vi "PV General operating info.vi"(8 "error in (no error)":errorcluster, 9 "Parameter":u16(ring) items=["nominal speed [Hz] (default) (315)", "intermediate circut current [A] (310)", "motor voltage [V] (313)", "actual power [W] (316)", "operating hours pump [h] (311)", "operating hours drive [h] (314)", "pump cycles (read only) (319)", "status oil sensor (read only) (301)", "speed switchpoint attained (read only) (302)", "overtemperature drive (read only) (304)", "overtemperature pump (read only) (305)", "target speed attained (read only) (306)", "pump accelerates (read only) (307) ", "controlled by remote (300)", "motor phase current [A] (317)", "acceleration / deceleration [rm/s] (336)", "hardware version controller (354)", "target speed (397)", "acutal speed (398)", "nominal speed (399)", "software version control unit (read only) (352)"], 10 "Adress of unit":u16=1 min=1 max=999 step=1, 11 "VISA session":refnum<visa-resource-name>) -> (0 "error out":errorcluster, 2 "response (data)":string, 3 "dup VISA session":refnum<visa-resource-name>)   [LabVIEW 2018, in "Pfeiffer Vacuum.lvlib"]
doc: "There are 21 parameters available, only one of which can be enabled at a time. \n\nnominal speed [Hz] (default) (315)\nintermediate circut current [A] (310)\nmotor voltage [V] (313)\nactual power [W] (316)\noperating hours pump [h] (311)\noperating hours drive [h] (314)\npump cycles (read only) (319)\nstatus oil sensor (read only) (301)\nspeed switchpoint attained (read only) (302)\novertemperature drive (read only) (304)\novertemperature pump (read only) (305)\ntarget speed attained (read only) (306)\npump accelerates (read only) (307)\ncontrolled by remote (300)\nmotor phase current [A] (317)\nacceleration / deceleration [rm/s] (336)\nhardware version controller (354)\ntarget speed (397)\nacutal speed (398)\nnominal speed (399)\nsoftware version control unit (read only) (352)\n\nNote: read only VI´s"
uses:
  Pfeiffer Vacuum.lvlib
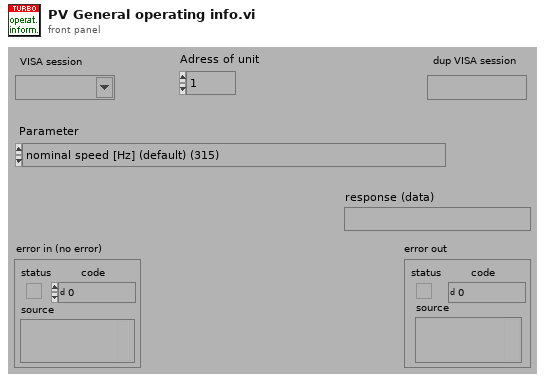
[diagram p1: front panel]
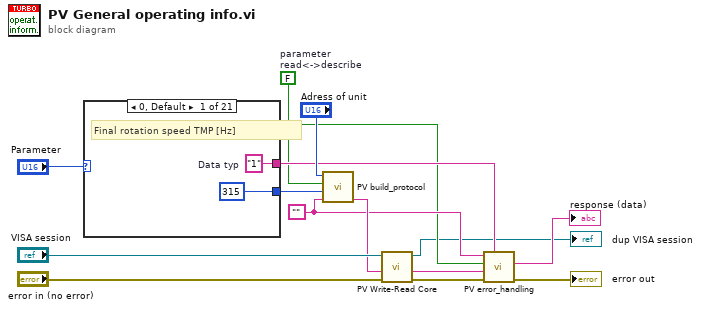
[diagram p0: block diagram]
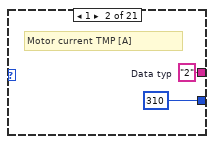
[diagram p2: hidden frame]
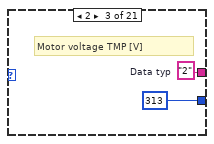
[diagram p3: hidden frame]
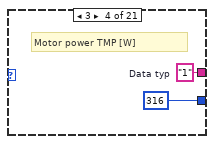
[diagram p4: hidden frame]
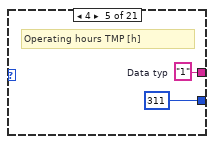
[diagram p5: hidden frame]
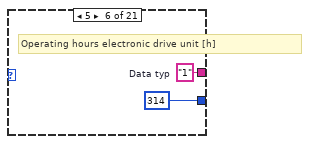
[diagram p6: hidden frame]
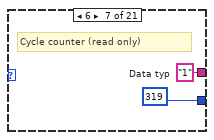
[diagram p7: hidden frame]
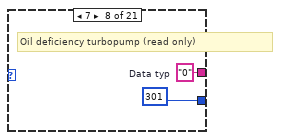
[diagram p8: hidden frame]
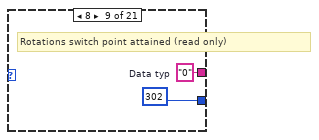
[diagram p9: hidden frame]
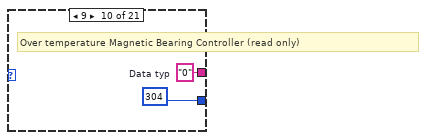
[diagram p10: hidden frame]
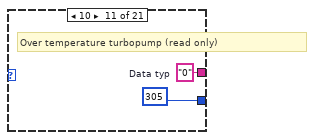
[diagram p11: hidden frame]
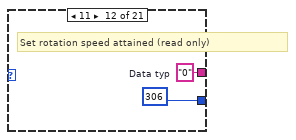
[diagram p12: hidden frame]
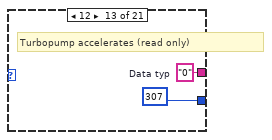
[diagram p13: hidden frame]
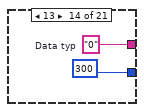
[diagram p14: hidden frame]
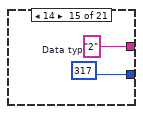
[diagram p15: hidden frame]
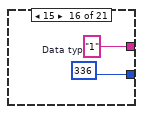
[diagram p16: hidden frame]
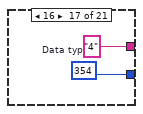
[diagram p17: hidden frame]
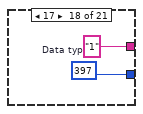
[diagram p18: hidden frame]
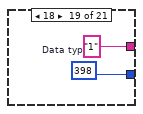
[diagram p19: hidden frame]
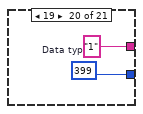
[diagram p20: hidden frame]
diagram:
  w7 = ""
  w6 = FALSE  # parameter read<->describe
  n1 = case shown="0, Default" "Parameter" {
    tunnel: [u16 315 ("Parameter-number") u16 310 ("Parameter-number") u16 313 ("Parameter-number") u16 316 ("Parameter-number") u16 311 ("Parameter-number") u16 314 ("Parameter-number") 319 301 302 304 305 306 307 300 317 336 354 397 398 399 352] -> w12
    tunnel: [w15 w17 w19 w21 w23 w25 w27 w29 w31 w33 w35 w37 w39 w41 w43 w45 w47 w49 w51 w53 w55] -> w8
    frame 0, Default {
      w15 = "1"  # Data typ
      # "Final rotation speed TMP [Hz]"
    }
    frame 1 {
      w17 = "2"  # Data typ
      # "Motor current TMP [A]"
    }
    frame 2 {
      w19 = "2"  # Data typ
      # "Motor voltage TMP [V]"
    }
    frame 3 {
      w21 = "1"  # Data typ
      # "Motor power TMP [W]"
    }
    frame 4 {
      w23 = "1"  # Data typ
      # "Operating hours TMP [h]"
    }
    frame 5 {
      w25 = "1"  # Data typ
      # "Operating hours electronic drive unit [h]"
    }
    frame 6 {
      w27 = "1"  # Data typ
      # "Cycle counter (read only)"
    }
    frame 7 {
      w29 = "0"  # Data typ
      # "Oil deficiency turbopump (read only)"
    }
    frame 8 {
      w31 = "0"  # Data typ
      # "Rotations switch point attained (read only)"
    }
    frame 9 {
      w33 = "0"  # Data typ
      # "Over temperature Magnetic Bearing Controller (read only)"
    }
    frame 10 {
      w35 = "0"  # Data typ
      # "Over temperature turbopump (read only)"
    }
    frame 11 {
      w37 = "0"  # Data typ
      # "Set rotation speed attained (read only)"
    }
    frame 12 {
      w39 = "0"  # Data typ
      # "Turbopump accelerates (read only)"
    }
    frame 13 {
      w41 = "0"  # Data typ
    }
    frame 14 {
      w43 = "2"  # Data typ
    }
    frame 15 {
      w45 = "1"  # Data typ
    }
    frame 16 {
      w47 = "4"  # Data typ
    }
    frame 17 {
      w49 = "1"  # Data typ
    }
    frame 18 {
      w51 = "1"  # Data typ
    }
    frame 19 {
      w53 = "1"  # Data typ
    }
    frame 20 {
      w55 = "4"  # Data typ
    }
  }
  n2 = call "PV build_protocol.vi"("Data"=w7, "Parameter-number"=w12, "parameter\nread<->describe"=w6, "Adress"="Adress of unit") -> ("output"=w9:string)  [unwired: 3 in]
  n3 = call "PV Write-Read Core.vi"("error in"="error in (no error)", "Write data in"=w9, "VISA session"="VISA session") -> ("error out"=w4:errorcluster, "response (data) out"=w5:string, "dup VISA session"=→"dup VISA session":refnum<visa-resource-name>)  [unwired: 2 in]
  n4 = call "PV error_handling.vi"("Data Typ in"=w8, "error in"=w4, "response (data) in"=w5, "Parameter\nread only<->describe"=w6, "data in"=w7) -> ("error out"=→"error out":errorcluster, "Data out"=→"response (data)":string)  [unwired: 4 in, 1 out]
